vi "Timer.vi"(8 "error in":errorcluster, 10 "Time Target":dbl=7.0, 11 "Timer Mode":T1) -> (0 "error out":errorcluster, 2 "Time Has Elapsed":bool, 3 "Elapsed Time (s)":dbl)   [LabVIEW 2018]
doc: "This Vi counts the time and implements a pause routine"
uses:
  Controls/Timer Mode.ctl
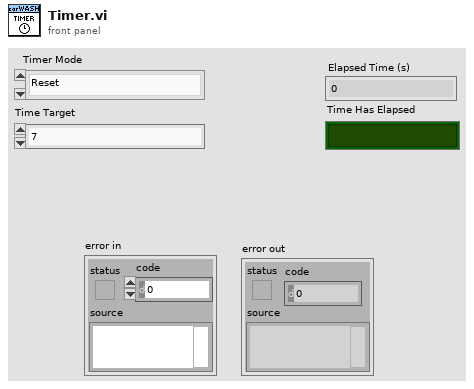
[diagram p1: front panel]
types:
  T1 = typedef "Timer Mode.ctl" = enum16{"Reset", "Get Time", "Start", "Pause"}
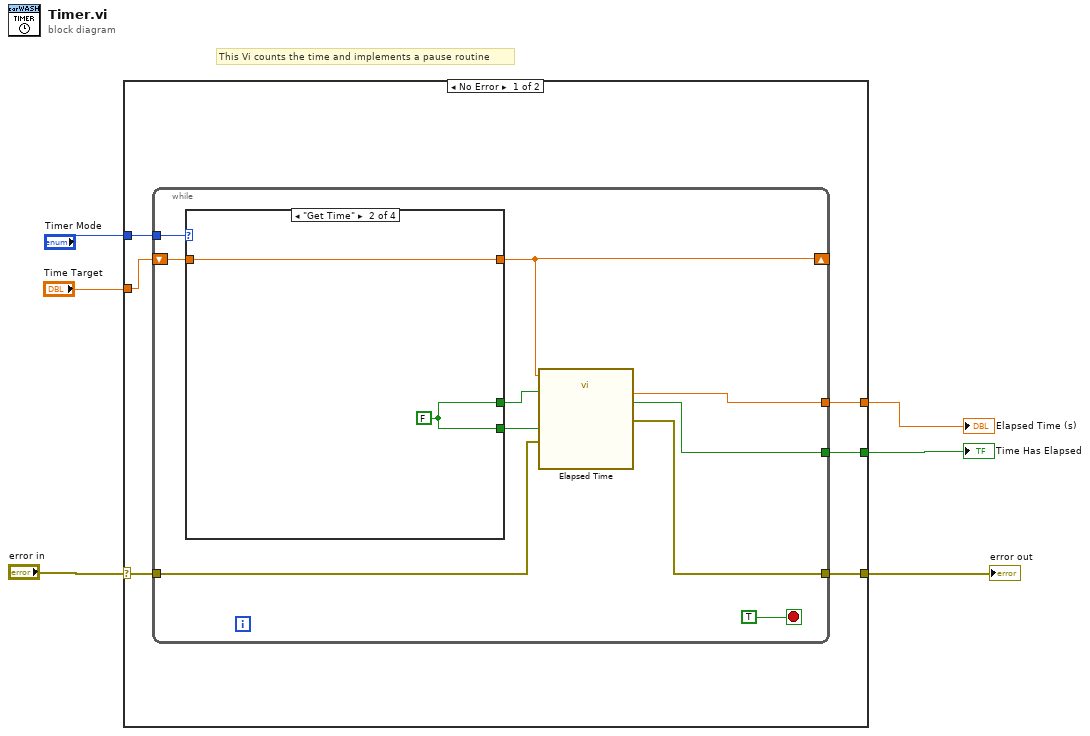
[diagram p0: block diagram]
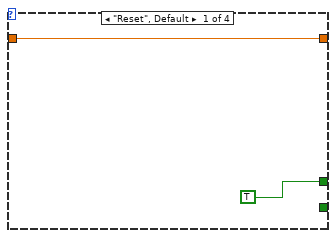
[diagram p2: hidden frame]
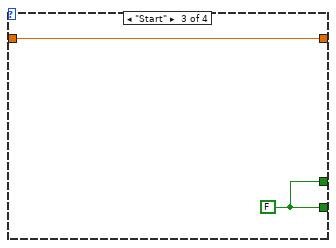
[diagram p3: hidden frame]
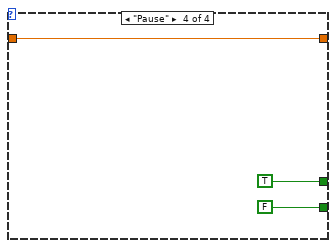
[diagram p4: hidden frame]
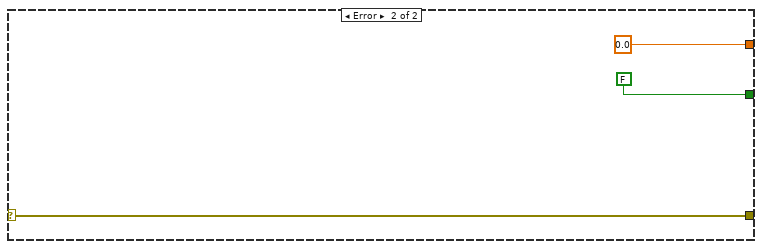
[diagram p5: hidden frame]
diagram:
  # "This Vi counts the time and implements a pause routine"
  n1 = case shown="No Error" "error in" {
    selector: "error in" -> [w9 w34]
    tunnel: [w8 w34] -> w5
    tunnel: "Timer Mode" -> [w12 _]
    tunnel: "Time Target" -> [w7 _]
    tunnel: [w11 0.0 ("Elapsed Time (s)")] -> w3
    tunnel: [w10 FALSE ("Time has Elapsed")] -> w2
    frame No Error {
      n2 = while {
        tunnel: w12 -> [w22]
        tunnel: [w20] -> w11
        tunnel: [w19] -> w10
        shift-right: [w17] -> _
        shift-left: w7 -> [w18]
        tunnel: w9 -> [w14]
        tunnel: [w16] -> w8
        stop <- TRUE stop-if-true
        n3 = case shown="\"Get Time\"" w22 {
          tunnel: [TRUE w25 w28 TRUE] -> w21
          tunnel: [w23 w26 w27 w31] -> w17
          tunnel: w18 -> [w23 w26 w27 w31]
          tunnel: [_ w25 w28 FALSE] -> w13
          frame "Reset", Default {
          }
          frame "Get Time" {
            w25 = FALSE
          }
          frame "Start" {
            w28 = FALSE
          }
          frame "Pause" {
          }
        }
        n4 = call "Elapsed Time"("Time Target (s)"=w17, "Reset"=w21, "Auto Reset"=w13, "error in (no error)"=w14) -> ("Elapsed Time (s)"=w20:dbl, "Time has Elapsed"=w19:bool, "error out"=w16:errorcluster)  [unwired: 8 in, 5 out]
      }
    }
    frame Error {
    }
  }
  "error out" <- w5
  "Elapsed Time (s)" <- w3
  "Time Has Elapsed" <- w2
